vi "25-15-5-2.vi"() -> ()   [LabVIEW 2025]
uses:
  <vilib>/Platform/TimedLoop/XDataNode/timing_clust.ctl
  <vilib>/Platform/TimedLoop/XDataNode/nitl_modes.ctl
  <vilib>/Platform/TimedLoop/XDataNode/wakeup.ctl
  <vilib>/rvi/Emulation/niFpgaSctlEmulationGetInTimedLoop.vi
  <vilib>/rvi/Emulation/niFpgaEmulationReportErrorSimple.vi
  <vilib>/rvi/Emulation/niFpgaGetClockAttributes.vi
  <vilib>/rvi/Emulation/niFpgaCriticalErrorInLSC.vi
  <vilib>/rvi/linearAlgebra/MatrixMultiply/simVIs/SubVI/nifxpla_MatrixMultiply_SimMatrixSizes.vi
  <vilib>/rvi/linearAlgebra/MatrixMultiply/simVIs/SubVI/nifxpla_MatrixMultiply_Sim4WireAdapterVector.vi
  <vilib>/rvi/linearAlgebra/MatrixMultiply/simVIs/SubVI/nifxpla_MatrixMultiply_SimFrameHandShake.vi
  <vilib>/rvi/linearAlgebra/MatrixMultiply/simVIs/SubVI/nifxpla_MatrixMultiply_SimEndlessCounter.vi
  <vilib>/rvi/linearAlgebra/MatrixMultiply/simVIs/SubVI/nifxpla_MatrixMultiply_SimVectorDataBuffer.vi
  <vilib>/rvi/ClientSDK/Core/DevComputerLib/Private/Multiply(dfxp64).vi
  <vilib>/rvi/ClientSDK/Core/DevComputerLib/Private/Dfxp128ToDfxp256.vi
  <vilib>/rvi/ClientSDK/Core/DevComputerLib/Private/Add(dfxp256).vi
  <vilib>/rvi/ClientSDK/Core/DevComputerLib/Private/Subtract(dfxp256).vi
  <vilib>/rvi/ClientSDK/Core/DevComputerLib/Private/ToDfxp64(dfxp256).vi
  <vilib>/platform/TimedLoop/XDataNode/XDataNode.xnode
  <vilib>/rvi/linearAlgebra/MatrixMultiply/XNode/nifxpla_MatrixMultiply.xnode
  <vilib>/rvi/linearAlgebra/MatrixMultiply/simVIs/nifxpla_MatrixMultiply_SimTemplateEinEout.vi
  <vilib>/rvi/linearAlgebra/MatrixMultiply/simVIs/nifxpla_MatrixMultiply_SimTemplateEinVout.vi
  <vilib>/rvi/linearAlgebra/MatrixMultiply/simVIs/nifxpla_MatrixMultiply_SimTemplateVinEout.vi
  <vilib>/rvi/linearAlgebra/MatrixMultiply/simVIs/nifxpla_MatrixMultiply_SimTemplateVinVout.vi
  <vilib>/Platform/TimedLoop/XDataNode/XDNodeRunTimeDep.lvlib
panel:
  out "Latency":u32
  out "Cycle Count 3":i32
  out "C3":fxp<+/-,32,16>[](array[numeric])
  out "C3+B":fxp<+/-,33,17>[](array[numeric])
  out "Cycle Count 2":i32
  out "C2":fxp<+/-,32,16>[](array[numeric])
  out "C2+B":fxp<+/-,33,17>[](array[numeric])
  out "Cycle Count":i32
  out "C1":fxp<+/-,32,16>[](array[numeric])
  out "C1+B":fxp<+/-,33,17>[](array[numeric])
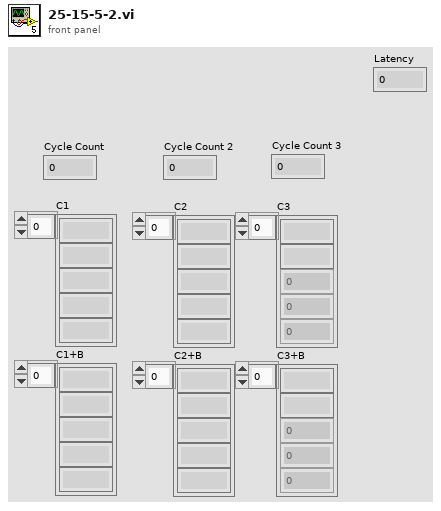
[diagram p1: front panel]
types:
  T1 = typedef "XDNodeRunTimeDep.lvlib/timing_clust.ctl" = cluster{"Expected End [f-1]":u64, "Actual End [f-1]":u64, "Finished Late? [f-1]":bool, "Expected End [i-1]":u64, "Actual End [i-1]":u64, "Finished Late? [i-1]":bool, "Expected Start [i]":u64, "Actual Start [i]":u64, "Expected Start [f]":u64, "Actual Start [f]":u64, "Source Name":string, "Structure Name":string, "Period":i64, "Deadline":i64, "Offset":i64, "Start":i64, "Priority":i32, "Timeout":i32, "Mode":T2, "Wakeup Reason":T3, "Error":errorcluster, "Source Type":string, "Secondary Source Type":string, "Global End Time":u64, "Global Start Time":u64, "Frame Duration":u64, "Iteration Duration":u64, "Assigned CPU":i32, "I/O Scan Engine Mode":u32}
  T2 = typedef "XDNodeRunTimeDep.lvlib/nitl_modes.ctl" = enum32{"No Change", "Process missed periods, maintain original phase", "Discard missed periods, maintain original phase", "Process missed periods, ignore original phase", "Discard missed periods, ignore original phase"}
  T3 = typedef "XDNodeRunTimeDep.lvlib/wakeup.ctl" = enum32{"Normal", "Aborted", "Asynchronous wakeup", "Timing source error", "Timed loop error", "Timeout"}
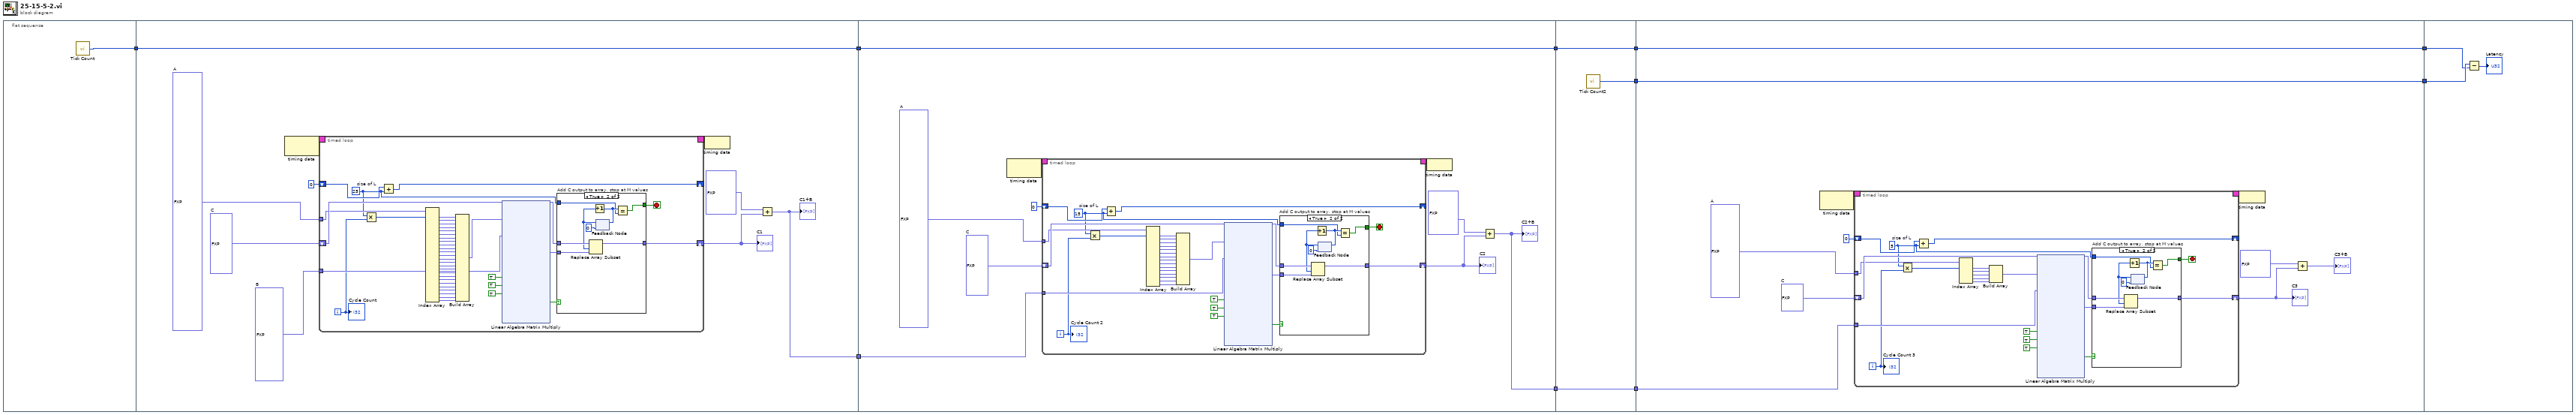
[diagram p0: block diagram]
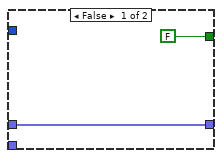
[diagram p2: hidden frame]
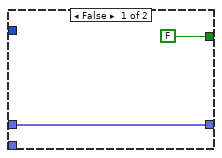
[diagram p3: hidden frame]
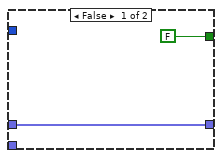
[diagram p4: hidden frame]
diagram:
  n1 = flat-sequence {
    tunnel: [w11] -> w10
    tunnel: [w13] -> w9
    tunnel: [w12] -> w8
    tunnel: w10 -> [w12]
    tunnel: w9 -> [w80]
    tunnel: [w79] -> w7
    tunnel: w8 -> [w78]
    tunnel: [w78] -> w6
    tunnel: w7 -> [w134]
    tunnel: [w134] -> w5
    tunnel: w6 -> [w133]
    tunnel: [w133] -> w4
    tunnel: [w132] -> w3
    tunnel: w5 -> [w137]
    tunnel: w4 -> [w136]
    tunnel: [w136] -> w2
    tunnel: [w135] -> w1
    tunnel: w3 -> [w135]
    tunnel: w2 -> [w182]
    tunnel: w1 -> [w183]
    frame #0 {
      n2 = call "Tick Count"() -> ("Tick Count(Ticks)"=w11:u32)
    }
    frame #1 {
      w17 = fxp<+/-,32,16>[] [0.0, 0.0, 0.0, 0.0, 0.0, 0.0, 0.0, 0.0, 0.0, 0.0, 0.0, 0.0, 0.0, 0.0, 0.0, 0.0, 0.0, 0.0, 0.0, 0.0, 0.0, 0.0, 0.0, 0.0, 0.0, 0.0, 0.0, 0.0, 0.0, 0.0, 0.0, 0.0, 0.0, 0.0, 0.0, 0.0, 0.0, 0.0, 0.0, 0.0, 0.0, 0.0, 0.0, 0.0, 0.0, 0.0, 0.0, 0.0, 0.0, 0.0, 0.0, 0.0, 0.0, 0.0, 0.0, 0.0, 0.0, 0.0, 0.0, 0.0, 0.0, 0.0, 0.0, 0.0, 0.0, 0.0, 0.0, 0.0, 0.0, 0.0, 0.0, 0.0, 0.0, 0.0, 0.0, 0.0, 0.0, 0.0, 0.0, 0.0, 0.0, 0.0, 0.0, 0.0, 0.0, 0.0, 0.0, 0.0, 0.0, 0.0, 0.0, 0.0, 0.0, 0.0, 0.0, 0.0, 0.0, 0.0, 0.0, 0.0, 0.0, 0.0, 0.0, 0.0, 0.0, 0.0, 0.0, 0.0, 0.0, 0.0, 0.0, 0.0, 0.0, 0.0, 0.0, 0.0, 0.0, 0.0, 0.0, 0.0, 0.0, 0.0, 0.0, 0.0, 0.0, 0.0, 0.0, 0.0, 0.0, 0.0, 0.0, 0.0, 0.0, 0.0, 0.0, 0.0, 0.0, 0.0, 0.0, 0.0, 0.0, 0.0, 0.0, 0.0, 0.0, 0.0, 0.0, 0.0, 0.0, 0.0, 0.0, 0.0, 0.0, 0.0, 0.0, 0.0, 0.0, 0.0, 0.0, 0.0, 0.0, 0.0, 0.0, 0.0, 0.0, 0.0, 0.0, 0.0, 0.0, 0.0, 0.0, 0.0, 0.0, 0.0, 0.0, 0.0, 0.0, 0.0, 0.0, 0.0, 0.0, 0.0, 0.0, 0.0, 0.0, 0.0, 0.0, 0.0, 0.0, 0.0, 0.0, 0.0, 0.0, 0.0, 0.0, 0.0, 0.0, 0.0, 0.0, 0.0, 0.0, 0.0, 0.0, 0.0, 0.0, 0.0, 0.0, 0.0, 0.0, 0.0, 0.0, 0.0, 0.0, 0.0, 0.0, 0.0, 0.0, 0.0, 0.0, 0.0, 0.0, 0.0, 0.0, 0.0, 0.0, 0.0, 0.0, 0.0, 0.0, 0.0, 0.0, 0.0, 0.0, 0.0, 0.0, 0.0, 0.0, 0.0, 0.0, 0.0, 0.0, 0.0, 0.0, 0.0, 0.0, 0.0, 0.0, 0.0, 0.0, 0.0, 0.0, 0.0, 0.0, 0.0, 0.0, 0.0, 0.0, 0.0, 0.0, 0.0, 0.0, 0.0, 0.0, 0.0, 0.0, 0.0, 0.0, 0.0, 0.0, 0.0, 0.0, 0.0, 0.0, 0.0, 0.0, 0.0, 0.0, 0.0, 0.0, 0.0, 0.0, 0.0, 0.0, 0.0, 0.0, 0.0, 0.0, 0.0, 0.0, 0.0, 0.0, 0.0, 0.0, 0.0, 0.0, 0.0, 0.0, 0.0, 0.0, 0.0, 0.0, 0.0, 0.0, 0.0, 0.0, 0.0, 0.0, 0.0, 0.0, 0.0, 0.0, 0.0, 0.0, 0.0, 0.0, 0.0, 0.0, 0.0, 0.0, 0.0, 0.0, 0.0, 0.0, 0.0, 0.0, 0.0, 0.0, 0.0, 0.0, 0.0, 0.0, 0.0, 0.0, 0.0, 0.0, 0.0, 0.0, 0.0, 0.0, 0.0, 0.0, 0.0, 0.0, 0.0, 0.0, 0.0, 0.0, 0.0, 0.0, 0.0, 0.0, 0.0, 0.0, 0.0, 0.0, 0.0, 0.0, 0.0, 0.0, 0.0, 0.0, 0.0, 0.0, 0.0, 0.0, 0.0, 0.0, 0.0, 0.0, 0.0, 0.0, 0.0, 0.0, 0.0, 0.0]  # A
      w18 = fxp<+/-,32,16>[] [0.0, 0.0, 0.0, 0.0, 0.0, 0.0, 0.0, 0.0, 0.0, 0.0, 0.0, 0.0, 0.0, 0.0, 0.0, 0.0, 0.0, 0.0, 0.0, 0.0, 0.0, 0.0, 0.0, 0.0, 0.0]  # B
      w19 = fxp<+/-,32,16>[] [0.0, 0.0, 0.0, 0.0, 0.0, 0.0, 0.0, 0.0, 0.0, 0.0, 0.0, 0.0, 0.0, 0.0, 0.0]  # C
      n3 = node-c288() -> (w21:T1)  [unwired: 1 in]
      n4 = timed-loop {
        timing: w21 -> [_]
        timing-out: [_] -> w20
        shift-right: [w61] -> w15
        shift-left: w19 -> [w60]
        tunnel: w18 -> [w57]
        tunnel: w17 -> [w40]
        shift-right: [w53] -> _
        shift-left: 0 ("length") -> [w54]
        i -> [w39]
        stop <- w59 stop-if-true
        w38 = 25  # size of L
        n5 = Multiply(x=w38, y=w39) -> (x*y=w51:i32)
        n6 = Add(x=w54, y=w38) -> (x+y=w53:i32)
        n7 = Index Array(array=w40, index #1=w51) -> (element #1=w50:fxp<+/-,32,16>, element #2=w49:fxp<+/-,32,16>, element #3=w48:fxp<+/-,32,16>, element #4=w47:fxp<+/-,32,16>, element #5=w46:fxp<+/-,32,16>, element #6=w45:fxp<+/-,32,16>, element #7=w44:fxp<+/-,32,16>, element #8=w43:fxp<+/-,32,16>, element #9=w42:fxp<+/-,32,16>, element #10=w41:fxp<+/-,32,16>, element #11=w36:fxp<+/-,32,16>, element #12=w35:fxp<+/-,32,16>, element #13=w34:fxp<+/-,32,16>, element #14=w33:fxp<+/-,32,16>, element #15=w32:fxp<+/-,32,16>, element #16=w31:fxp<+/-,32,16>, element #17=w30:fxp<+/-,32,16>, element #18=w29:fxp<+/-,32,16>, element #19=w28:fxp<+/-,32,16>, element #20=w27:fxp<+/-,32,16>, element #21=w26:fxp<+/-,32,16>, element #22=w25:fxp<+/-,32,16>, element #23=w24:fxp<+/-,32,16>, element #24=w23:fxp<+/-,32,16>, element #25=w22:fxp<+/-,32,16>)  [unwired: 24 in]
        n8 = Build Array(w50, w49, w48, w47, w46, w45, w44, w43, w42, w41, w36, w35, w34, w33, w32, w31, w30, w29, w28, w27, w26, w25, w24, w23, w22) -> (w37:fxp<+/-,32,16>[])
        n9 = xnode ("Linear Algebra Matrix Multiply")("ar"=w37, "br"=w57, "a valid"=TRUE, "b valid"=TRUE, "ready for output (T)"=TRUE) -> ("cr"=w56:fxp<+/-,64,37>[], "output valid"=w52:bool)  [unwired: 2 in, 4 out]
        n10 = case "Add C output to array, stop at M values" shown="True" w52 {
          tunnel: w56 -> [_ w68]
          tunnel: [w64 w71] -> w61
          tunnel: w60 -> [w64 w72]
          tunnel: [FALSE w69] -> w59
          tunnel: w38 -> [_ w65]
          frame False {
          }
          frame True {
            n11 = feedback #1(0 ("x")) -> (w67:i32)
            n12 = Replace Array Subset(array=w72, new element=w68, index=w67) -> (w71:fxp<+/-,32,16>[])
            n13 = Increment(x=w67) -> (x+1=w66:i32)
            n14 = feedback-in #1(w66) -> ()
            n15 = Equal?(x=w66, y=w65) -> (x = y?=w69:bool)
          }
        }
        "Cycle Count" <- w39
      }
      "C1" <- w15
      n16 = node-c288(w20) -> ()
      n17 = Add(x=fxp<+/-,32,16>[] [0.5, 0.5, 0.5, 0.5, 0.5, 0.0, 0.0, 0.0, 0.0, 0.0, 0.0, 0.0, 0.0, 0.0, 0.0], y=w15) -> (x+y=w13:fxp<+/-,33,17>[])
      "C1+B" <- w13
    }
    frame #2 {
      w83 = fxp<+/-,32,16>[] [0.0, 0.0, 0.0, 0.0, 0.0, 0.0, 0.0, 0.0, 0.0, 0.0, 0.0, 0.0, 0.0, 0.0, 0.0, 0.0, 0.0, 0.0, 0.0, 0.0, 0.0, 0.0, 0.0, 0.0, 0.0, 0.0, 0.0, 0.0, 0.0, 0.0, 0.0, 0.0, 0.0, 0.0, 0.0, 0.0, 0.0, 0.0, 0.0, 0.0, 0.0, 0.0, 0.0, 0.0, 0.0, 0.0, 0.0, 0.0, 0.0, 0.0, 0.0, 0.0, 0.0, 0.0, 0.0, 0.0, 0.0, 0.0, 0.0, 0.0, 0.0, 0.0, 0.0, 0.0, 0.0, 0.0, 0.0, 0.0, 0.0, 0.0, 0.0, 0.0, 0.0, 0.0, 0.0]  # A
      w84 = fxp<+/-,32,16>[] [0.0, 0.0, 0.0, 0.0, 0.0]  # C
      n18 = node-c288() -> (w86:T1)  [unwired: 1 in]
      n19 = timed-loop {
        timing: w86 -> [_]
        timing-out: [_] -> w85
        shift-right: [w116] -> w81
        shift-left: w84 -> [w115]
        tunnel: w80 -> [w112]
        tunnel: w83 -> [w100]
        shift-right: [w108] -> _
        shift-left: 0 ("length") -> [w109]
        i -> [w99]
        stop <- w114 stop-if-true
        w98 = 15  # size of L
        n20 = Multiply(x=w98, y=w99) -> (x*y=w106:i32)
        n21 = Add(x=w109, y=w98) -> (x+y=w108:i32)
        n22 = Index Array(array=w100, index #1=w106) -> (element #1=w105:fxp<+/-,32,16>, element #2=w104:fxp<+/-,32,16>, element #3=w103:fxp<+/-,32,16>, element #4=w102:fxp<+/-,32,16>, element #5=w101:fxp<+/-,32,16>, element #6=w96:fxp<+/-,32,16>, element #7=w95:fxp<+/-,32,16>, element #8=w94:fxp<+/-,32,16>, element #9=w93:fxp<+/-,32,16>, element #10=w92:fxp<+/-,32,16>, element #11=w91:fxp<+/-,32,16>, element #12=w90:fxp<+/-,32,16>, element #13=w89:fxp<+/-,32,16>, element #14=w88:fxp<+/-,32,16>, element #15=w87:fxp<+/-,32,16>)  [unwired: 14 in]
        n23 = Build Array(w105, w104, w103, w102, w101, w96, w95, w94, w93, w92, w91, w90, w89, w88, w87) -> (w97:fxp<+/-,32,16>[])
        n24 = xnode ("Linear Algebra Matrix Multiply")("ar"=w97, "br"=w112, "a valid"=TRUE, "b valid"=TRUE, "ready for output (T)"=TRUE) -> ("cr"=w111:fxp<+/-,64,37>[], "output valid"=w107:bool)  [unwired: 2 in, 4 out]
        n25 = case "Add C output to array, stop at M values" shown="True" w107 {
          tunnel: w111 -> [_ w123]
          tunnel: [w119 w126] -> w116
          tunnel: w115 -> [w119 w127]
          tunnel: [FALSE w124] -> w114
          tunnel: w98 -> [_ w120]
          frame False {
          }
          frame True {
            n26 = feedback #2(0 ("x")) -> (w122:i32)
            n27 = Replace Array Subset(array=w127, new element=w123, index=w122) -> (w126:fxp<+/-,32,16>[])
            n28 = Increment(x=w122) -> (x+1=w121:i32)
            n29 = feedback-in #2(w121) -> ()
            n30 = Equal?(x=w121, y=w120) -> (x = y?=w124:bool)
          }
        }
        "Cycle Count 2" <- w99
      }
      "C2" <- w81
      n31 = node-c288(w85) -> ()
      n32 = Add(x=fxp<+/-,32,16>[] [0.5, 0.5, 0.5, 0.5, 0.5], y=w81) -> (x+y=w79:fxp<+/-,33,17>[])
      "C2+B" <- w79
    }
    frame #3 {
      n33 = call "Tick Count2"() -> ("Tick Count(Ticks)"=w132:u32)
    }
    frame #4 {
      w142 = fxp<+/-,32,16>[] [0.0, 0.0, 0.0, 0.0, 0.0, 0.0, 0.0, 0.0, 0.0, 0.0]  # A
      w143 = fxp<+/-,32,16>[] [0.0, 0.0]  # C
      n34 = node-c288() -> (w145:T1)  [unwired: 1 in]
      n35 = timed-loop {
        timing: w145 -> [_]
        timing-out: [_] -> w144
        shift-right: [w165] -> w140
        shift-left: w143 -> [w164]
        tunnel: w137 -> [w161]
        tunnel: w142 -> [w149]
        shift-right: [w157] -> _
        shift-left: 0 ("length") -> [w158]
        i -> [w148]
        stop <- w163 stop-if-true
        w147 = 5  # size of L
        n36 = Multiply(x=w147, y=w148) -> (x*y=w155:i32)
        n37 = Add(x=w158, y=w147) -> (x+y=w157:i32)
        n38 = Index Array(array=w149, index #1=w155) -> (element #1=w154:fxp<+/-,32,16>, element #2=w153:fxp<+/-,32,16>, element #3=w152:fxp<+/-,32,16>, element #4=w151:fxp<+/-,32,16>, element #5=w150:fxp<+/-,32,16>)  [unwired: 4 in]
        n39 = Build Array(w154, w153, w152, w151, w150) -> (w146:fxp<+/-,32,16>[])
        n40 = xnode ("Linear Algebra Matrix Multiply")("ar"=w146, "br"=w161, "a valid"=TRUE, "b valid"=TRUE, "ready for output (T)"=TRUE) -> ("cr"=w160:fxp<+/-,64,36>[], "output valid"=w156:bool)  [unwired: 2 in, 4 out]
        n41 = case "Add C output to array, stop at M values" shown="True" w156 {
          tunnel: w160 -> [_ w172]
          tunnel: [w168 w175] -> w165
          tunnel: w164 -> [w168 w176]
          tunnel: [FALSE w173] -> w163
          tunnel: w147 -> [_ w169]
          frame False {
          }
          frame True {
            n42 = feedback #3(0 ("x")) -> (w171:i32)
            n43 = Replace Array Subset(array=w176, new element=w172, index=w171) -> (w175:fxp<+/-,32,16>[])
            n44 = Increment(x=w171) -> (x+1=w170:i32)
            n45 = feedback-in #3(w170) -> ()
            n46 = Equal?(x=w170, y=w169) -> (x = y?=w173:bool)
          }
        }
        "Cycle Count 3" <- w148
      }
      "C3" <- w140
      n47 = node-c288(w144) -> ()
      n48 = Add(x=fxp<+/-,32,16>[] [0.5, 0.5], y=w140) -> (x+y=→"C3+B":fxp<+/-,33,17>[])
    }
    frame #5 {
      n49 = Subtract(x=w183, y=w182) -> (x-y=→"Latency":u32)
    }
  }
